vi "Interpolate Spline.vi"(8 "time base":dbl[](array[numeric]) format="%_6g", 9 "X in":dbl[](array[numeric]), 10 "Y in":dbl[](array[numeric])) -> (2 "yi":dbl[](array[numeric]) format="%_6g")   [LabVIEW 2014]
uses:
  <vilib>/gmath/NI_Gmath.lvlib
panel:
  out "X in 2":dbl[](array[numeric])
  out "Y in 2":dbl[](array[numeric])
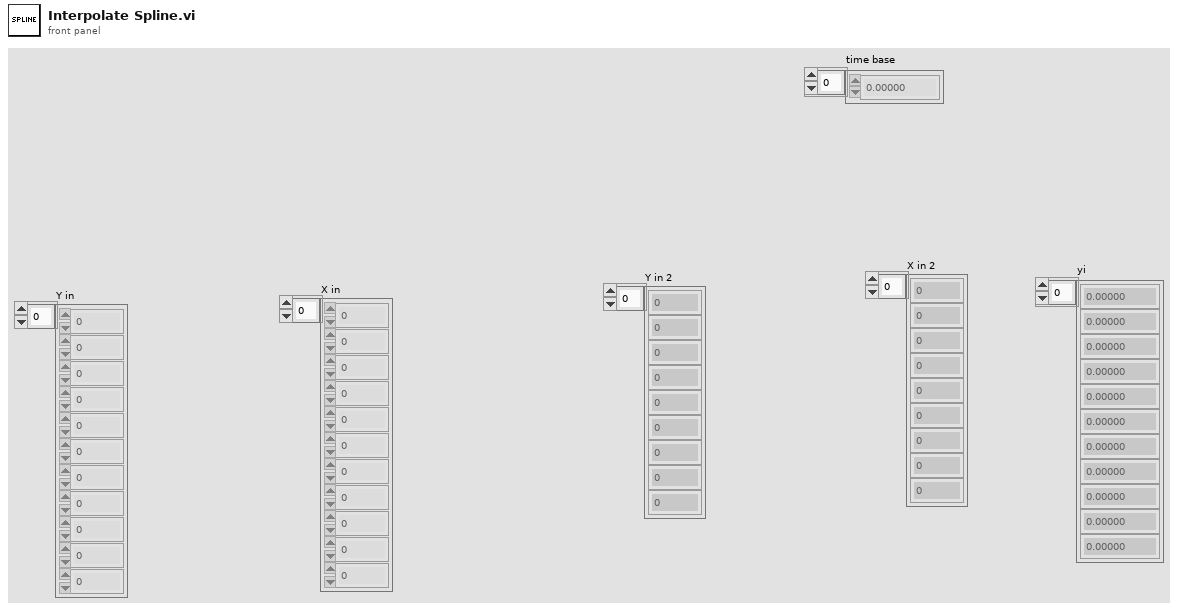
[diagram p1: front panel]
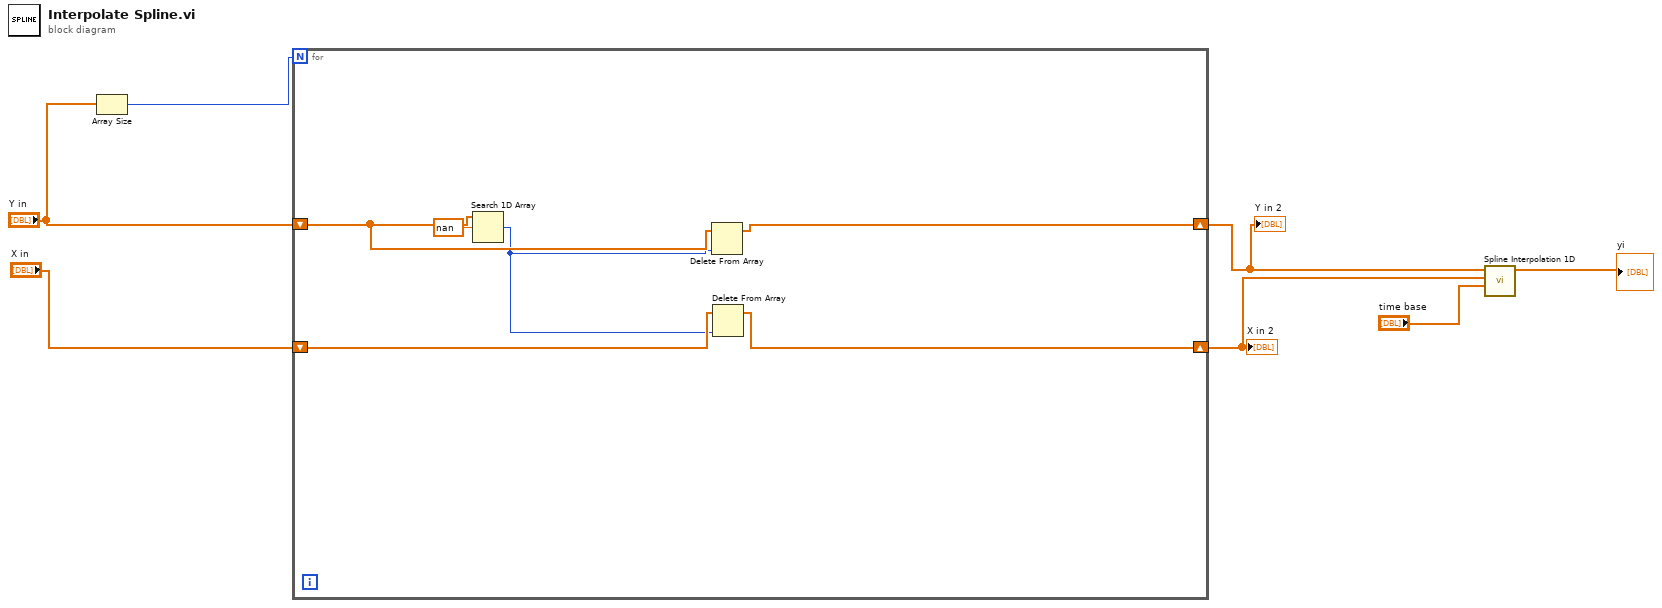
[diagram p0: block diagram]
diagram:
  n1 = Array Size(array="Y in") -> (size(s)=w7:i32)
  n2 = for {
    N: w7 -> [_]
    shift-right: [w9] -> w5
    shift-left: "Y in" -> [w12]
    shift-right: [w8] -> w4
    shift-left: "X in" -> [w11]
    n3 = Search 1D Array(1D array=w12, element=nan) -> (index of element=w10:i32)  [unwired: 1 in]
    n4 = Delete From Array(array=w12, index=w10) -> (array with subset deleted=w9:dbl[])  [unwired: 1 in, 1 out]
    n5 = Delete From Array(array=w11, index=w10) -> (array with subset deleted=w8:dbl[])  [unwired: 1 in, 1 out]
  }
  "Y in 2" <- w5
  "X in 2" <- w4
  n6 = call <vilib>:"Spline Interpolation 1D.vi"("xi"="time base", "X"=w4, "Y"=w5) -> ("yi"=→"yi":dbl[])  [unwired: 6 in, 2 out]
